vi "Save Configuration.vi"(8 "error in (no error)":errorcluster, 10 "File path":path, 11 "Monitor-Pulse in":refnum<class "LabActor.lvclass">) -> (0 "error out":errorcluster, 1 "Section out":string, 2 "File path out":path, 3 "Monitor-Pulse out":refnum<class "LabActor.lvclass">)   [LabVIEW 2018, in "LabActor.lvclass"]
uses:
  LabActor.lvclass
  C:/github/LabActor/Controllers/Application Controller/Application Controller.lvclass
  Controllers/Application Controller/Application Controller.lvclass/Application Controller.ctl
  LabActor.lvclass/LabActor.ctl
  Controllers/Application Controller/Read Postproc ref.vi
  NHMFL_Core/Libraries/Queued Listbox/Queued Listbox.xctl
  Controllers/Application Controller/Application Controller.lvclass
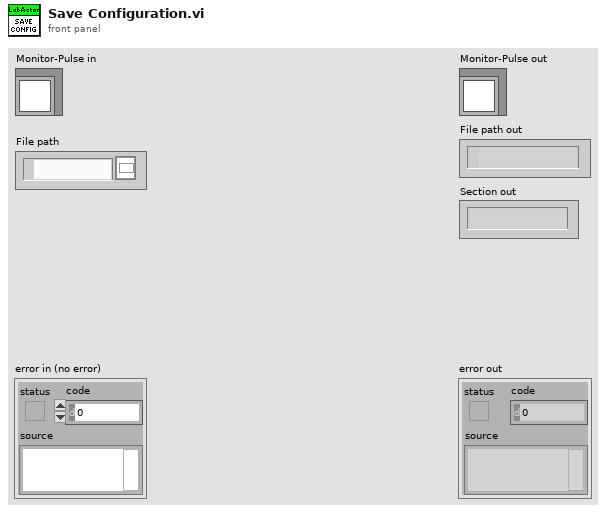
[diagram p1: front panel]
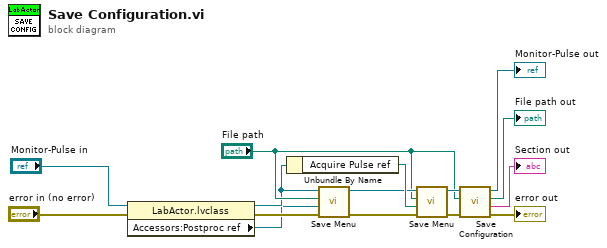
[diagram p0: block diagram]
diagram:
  n1 = property class="LabActor.lvclass"(reference="Monitor-Pulse in", error in="error in (no error)") -> (reference out=w2:refnum<class "LabActor.lvclass">, error out=w4:errorcluster, "Accessors:Postproc ref"=w1:refnum<vi>)
  n2 = Unbundle By Name(w2) -> ("Acquire Pulse ref"=w11:refnum<vi>)
  n3 = call-dynamic "Save Menu.vi"("error in (no error)"=w4, "Menu ref"=w1, "File path"="File path", "Monitor-Pulse in"=w2) -> ("error out"=w9:errorcluster, "Monitor-Pulse out"=w10:refnum<class "LabActor.lvclass">)  [unwired: 4 in, 2 out]
  n4 = call-dynamic "Save Menu.vi"("error in (no error)"=w9, "Menu ref"=w11, "File path"="File path", "Monitor-Pulse in"=w10) -> ("error out"=w7:errorcluster, "Monitor-Pulse out"=w6:refnum<class "LabActor.lvclass">)  [unwired: 4 in, 2 out]
  n5 = call-parent "Save Configuration.vi"("error in (no error)"=w7, "File path"="File path", "Measure Object in"=w6) -> ("error out"=→"error out":errorcluster, "Section out"=→"Section out":string, "File path out"=→"File path out":path, "Measure Object out"=→"Monitor-Pulse out":refnum<class "LabActor.lvclass">)  [unwired: 5 in]
